vi "Test proper PelcoD frame (SubVI).vi"(11 "Pelco-D frame":string) -> (3 "Proper?":bool)   [LabVIEW 2018]
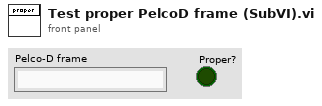
[diagram p1: front panel]
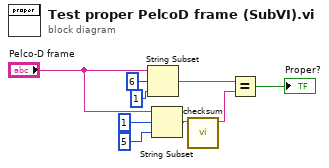
[diagram p0: block diagram]
diagram:
  n1 = String Subset(string="Pelco-D frame", offset (0)=6, length (rest)=1 ("length (rest)")) -> (substring=w7:string)
  n2 = String Subset(string="Pelco-D frame", offset (0)=1, length (rest)=5 ("length (rest)")) -> (substring=w3:string)
  n3 = call "checksum.vi"("msg"=w3) -> ("checksum"=w8:string)  [unwired: 10 in]
  n4 = Equal?(x=w7, y=w8) -> (x = y?=→"Proper?":bool)
